vi "Determine Script Strategy.vi"(10 "Template":string) -> (2 "Script Strategy":refnum<class "Script Strategy.lvclass">)   [LabVIEW 2021, in "_Template.lvlib" / "Script Strategy.lvlib"]
uses:
  Script Strategy.lvlib
  Script Strategy/Script Strategy.lvclass
  Msg Script Strategy/Msg Script Strategy.lvclass
  C:/git/jettl/tools/Template/_Template/Script Strategy/Script Strategy/Script Strategy.lvclass
  Actor Script Strategy/Actor Script Strategy.lvclass
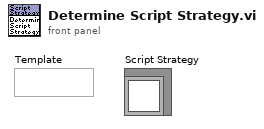
[diagram p1: front panel]
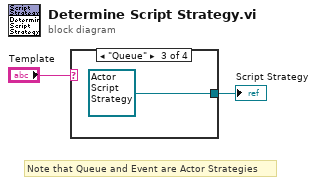
[diagram p0: block diagram]
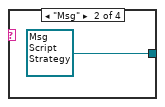
[diagram p3: hidden frame]
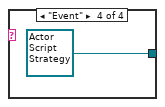
[diagram p4: hidden frame]
diagram:
  # "Note that Queue and Event are Actor Strategies"
  n1 = case shown="\"Queue\"" "Template" {
    tunnel: [_ refnum<class "Msg Script Strategy.lvclass"> refnum ("_Create From Template.lvlib:Script Strategy.lvlib:First Library Script Strategy.lvclass") refnum<class "Actor Script Strategy.lvclass"> refnum ("_Create From Template.lvlib:Script Strategy.lvlib:Actor Script Strategy.lvclass") refnum<class "Actor Script Strategy.lvclass"> refnum ("_Create From Template.lvlib:Script Strategy.lvlib:Second Library Script Strategy.lvclass")] -> w1
    frame Default {
    }
    frame "Msg" {
    }
    frame "Queue" {
    }
    frame "Event" {
    }
  }
  "Script Strategy" <- w1
